vi "ModelBLDC.vi"() -> ()   [LabVIEW 2018]
doc: "This example illustrates how to use six-step commutation to control the speed and rotation of a brushless DC motor.\n\nUnlike traditional DC motors, which are powered by mechanical commutation systems, brushless DC motors are powered by more reliable and more easily maintained electric commutation systems. In the six-step commutation method, the motor can have one of six combinations of on/off status, as determined by the rotor position, during one 360-degree electrical cycle."
uses:
  <vilib>/Simulation/Scripting/Companion Diagram/SimConfigNode/SimParams.ctl
  <vilib>/Simulation/Scripting/Companion Diagram/SimConfigNode/_simSolvers.ctl
  <vilib>/Simulation/Implementation/Shared/SIMSCR Execution Mode.ctl
  <vilib>/Simulation/Param Hierarchy/Typedefs/SIMPH Param Control Actions.ctl
  <vilib>/Simulation/Implementation/Shared/SIM limit type.ctl
  <vilib>/Simulation/Scripting/Editor Utilities/SIM subVI tag data.ctl
  <vilib>/Simulation/Scripting/Editor Utilities/SIM subVI execution type.ctl
  <vilib>/Simulation/Implementation/Shared/NILVSim_ParamChanged.vi
  <vilib>/Simulation/Implementation/Shared/NILVSIM_BeginStep.vi
  <vilib>/Simulation/Utility/Implementation/SIM Time.vi
  <vilib>/Simulation/Utility/Implementation/SIM Halt.vi
  <vilib>/Simulation/ContinuousLinear/Implementation/NILVSim Integrator new.llb/SIM Integrator distributor (scalar).vi
  <vilib>/Simulation/SignalDisplay/Implementation/NILVSim Time Waveform.llb/SIM Time Waveform (vector).vi
  <vilib>/Simulation/ContinuousLinear/Implementation/NILVSim Integrator new.llb/SIM Integrator collector (scalar).vi
  <vilib>/Simulation/Implementation/Shared/SIM Is Init or Final Stage.vi
  <vilib>/Simulation/Implementation/Shared/SIM Fire Discrete SubVI.vi
  <vilib>/Simulation/Implementation/Shared/NILVSim_Manager.vi
  <vilib>/Utility/error.llb/Clear Errors.vi
  <vilib>/Simulation/Implementation/Shared/NILVSim_FinalizeModel.vi
  <vilib>/Simulation/Implementation/Shared/SIM Fire Discrete SubVI (Core).vi
  <vilib>/Simulation/Implementation/Shared/SIM Unbundle Sim Info.vi
  <vilib>/Simulation/Implementation/Shared/NILVSim_Initialize.vi
  Program Files (x86)/National Instruments/LabVIEW 2018/examples/Control and Simulation/Case Studies/Electrical Machines/Brushless DC Motor Drive/subVIs/SimEx BLDC Animation.vi
  <vilib>/Simulation/Utility/Implementation/NILVSim Get Time and IsAcceptedStep.vi
  <vilib>/ptbypt/Other Functions.llb/Data Queue PtByPt.vi
  Program Files (x86)/National Instruments/LabVIEW 2018/examples/Control and Simulation/Case Studies/Electrical Machines/Brushless DC Motor Drive/subVIs/SimEx BLDC Hall Sensor.vi
  Program Files (x86)/National Instruments/LabVIEW 2018/examples/Control and Simulation/Case Studies/Electrical Machines/Brushless DC Motor Drive/subVIs/SimEx BLDC Six-step Controller.vi
  <vilib>/Simulation/Implementation/Shared/SIMSH Read Queue.vi
  <vilib>/Simulation/Implementation/Shared/NILVSim_GetModelError.vi
  <vilib>/Simulation/Implementation/Shared/SIM Bundle Sim Info.vi
  <vilib>/Simulation/Scripting/Companion Diagram/SimConfigNode/SimDog.xnode
  Program Files (x86)/National Instruments/LabVIEW 2018/examples/Control and Simulation/Case Studies/Electrical Machines/Brushless DC Motor Drive/SimEx Brushless DC Motor Drive Model.vi
  <vilib>/Simulation/Implementation/XNodeFramework/SimXNode/SimX.xnode
  <vilib>/ptbypt/NI_PtbyPt.lvlib
  <vilib>/Simulation/ContinuousLinear/Implementation/NILVSim Integrator new.llb/SIM Integrator (scalar).vi
  <vilib>/Simulation/Implementation/Shared/NI_SIM_Implementation.lvlib
panel:
  in  "Slow down simulation":bool=TRUE
  out "Motor Speed":dbl(knob)=86.1162484271292 scale=0.0..150.0
  in  "Mechanical Torque":dbl(slide)=3.8095238095238093 scale=0.0..10.0
  in  "Stop":bool
  in  "Tab Control":T1(tab)
  in  "BLDC Motor":enum32{"Mechanical ", "Electrical"}(tab)
  out "Hall C":bool
  out "Hall B":bool=TRUE
  out "Hall A":bool=TRUE
  out "BLCD Motor":picture
  out "Ib":dbl(knob)=17.922987920753645 scale=-100.0..100.0
  out "Ia":dbl(knob) scale=-100.0..100.0
  out "Ic":dbl(knob)=-17.734220639772992 scale=-100.0..100.0
  out "a hi":bool
  out "b hi":bool=TRUE
  out "c hi":bool
  out "b low":bool
  out "c low":bool=TRUE
  out "a low":bool
  out "Switch commutation":waveform(dbl)[](graph)=[{"t0"=timestamp(1.318615 s since 1904-01-01), "dt"=1.0, "Y"=[0.0]}, {"t0"=timestamp(1.318615 s since 1904-01-01), "dt"=1.0, "Y"=[1.0]}, {"t0"=timestamp(1.318615 s since 1904-01-01), "dt"=1.0, "Y"=[0.0]}, {"t0"=timestamp(1.318615 s since 1904-01-01), "dt"=1.0, "Y"=[0.0]}, {"t0"=timestamp(1.318615 s since 1904-01-01), "dt"=1.0, "Y"=[0.0]}, {"t0"=timestamp(1.318615 s since 1904-01-01), "dt"=1.0, "Y"=[1.0]}]
  in  "carrier frequency":dbl=10000.0
  in  "Vdc":dbl=25.0
  in  "duty cycle (0~1)":dbl=0.8
  out "Back EMF":waveform(dbl)[](graph)=[{"t0"=timestamp(1.318615 s since 1904-01-01), "dt"=1.0, "Y"=[0.23077392578125]}, {"t0"=timestamp(1.318615 s since 1904-01-01), "dt"=1.0, "Y"=[1.0]}, {"t0"=timestamp(1.318615 s since 1904-01-01), "dt"=1.0, "Y"=[-1.0]}]
  out "Current":waveform(dbl)[](graph)=[{"t0"=timestamp(1.318615 s since 1904-01-01), "dt"=1.0, "Y"=[0.0]}, {"t0"=timestamp(1.318615 s since 1904-01-01), "dt"=1.0, "Y"=[17.922987920753645]}, {"t0"=timestamp(1.318615 s since 1904-01-01), "dt"=1.0, "Y"=[-17.734220639772992]}]
  out "Speed (rad/s)":cluster{"Time":dbl[], "Signal":dbl[]}(graph)
  out "Ia (A)":cluster{"Time":dbl[], "Signal":dbl[]}(graph)
  out "Torque (N.m)":cluster{"Time":dbl[], "Signal":dbl[]}(graph)
  # "Overview: This example illustrates how to use six-step commutation to control the speed and rotation of a brushless DC motor. Unlike traditional DC motors, which are powered by mechanical commutation systems, brushless DC motors are powered by more reliable and more easily maintained electric commutation systems. In the six-step commutation method, the motor can have one of six combinations of on/off status, as determined by the rotor position, during one 360-degree electrical cycle.\nInstructions:\n1. Run the VI.\n2. Analyze the different signals from the simulatiuon by changing tabs. \n3. Change the mechanical Torque and see how that affect its speed."
  # "Vb"
  # "Va"
  # "Ia"
  # "Ib"
  # "Ic"
  # "Vc"
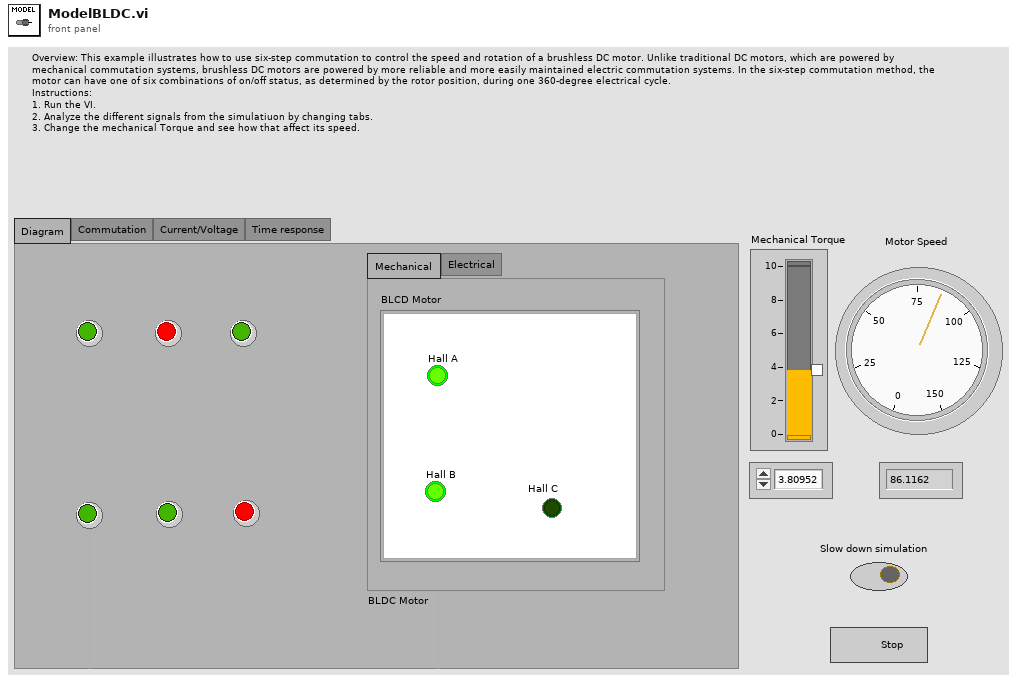
[diagram p1: front panel]
types:
  T1 = enum32{"Diagram", "Commutation", "Current/Voltage", "Time response"}
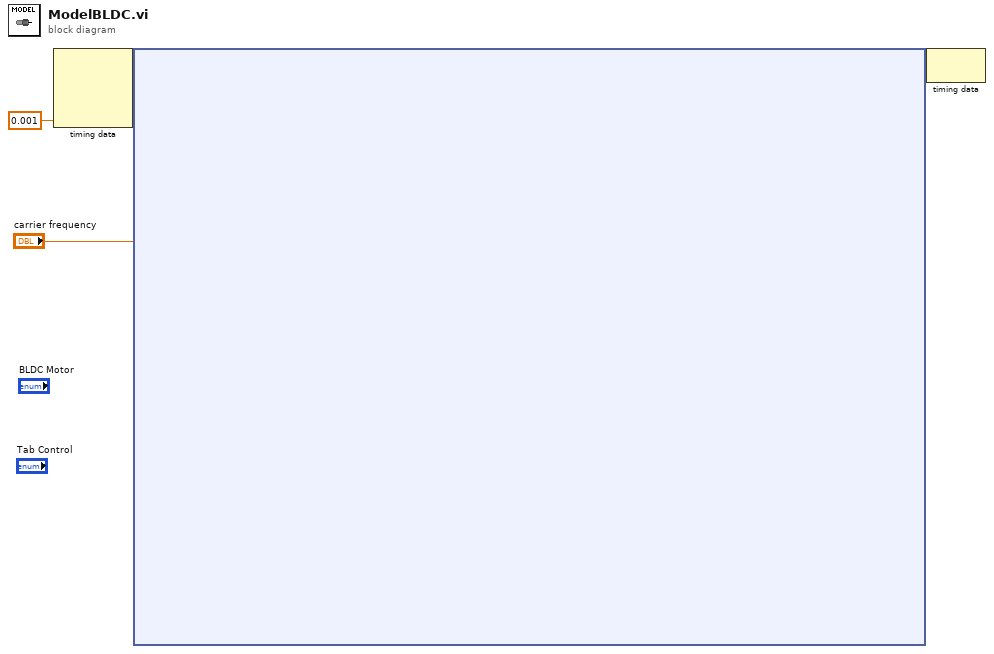
[diagram p0: block diagram]
diagram:
  n1 = node-c288(0.001 ("millisecond multiple")) -> (w4:variant)  [unwired: 3 out]
  n2 = node-c254 ("Simulation Loop")(w4, "carrier frequency") -> (w3:variant)
  n3 = node-c288(w3) -> ()  [unwired: 1 out]
